vi "Text as Encoded String (UTF-8 Path).vi"(9 "error in":errorcluster, 10 "Text":refnum<class "UTF-8 Path.lvclass">) -> (1 "error out":errorcluster, 2 "Encoded String":T1)   [LabVIEW 2020, in "G-Unicode.lvlib"]
doc: "Converts the input string or path to a raw UTF-8 encoded LabVIEW string. Valid inputs are a UTF-8 String class, UTF-8 Path class, LabVIEW string, or LabVIEW path."
uses:
  G-Unicode.lvlib
  Types/Encoded UTF-8 String.ctl
  Types/UTF-8 Path/UTF-8 Path.lvclass
  Types/UTF-8 Path/UTF-8 Path.lvclass/UTF-8 Path.ctl
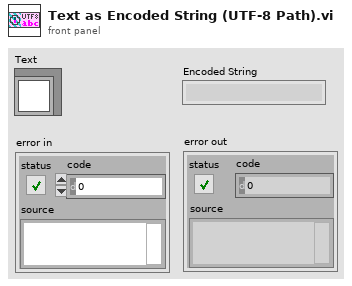
[diagram p1: front panel]
types:
  T1 = typedef "G-Unicode.lvlib/Encoded UTF-8 String.ctl" = string
  T2 = typedef "G-Unicode.lvlib/Encoded UTF-8 Path.ctl" = path
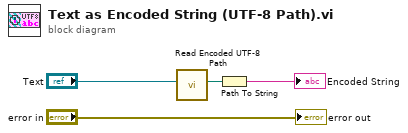
[diagram p0: block diagram]
diagram:
  n1 = call "Read Encoded UTF-8 Path.vi"("UTF-8 Path"="Text") -> ("Encoded UTF-8 Path"=w1:T2)  [unwired: 10 in]
  n2 = Path To String(path=w1) -> (string=→"Encoded String":string)
  "error out" <- "error in"
